vi "Test.vi"() -> ()   [LabVIEW 2014]
doc: "This VI is called when test mode begins, and will automatically be terminated when it ends. You can add manual or automatic tests and invoke them from the dashboard."
uses:
  <vilib>/Rock Robotics/WPI/RobotDrive/WPI_RobotDriveOpen2MotorWithTalon.vi
  <vilib>/Rock Robotics/SystemInterfaces/DIO/FPGA_DIOPWMChannel.ctl
  <vilib>/Rock Robotics/WPI/Joystick/WPI_JoystickDeviceEnum.ctl
panel:
  out "Distance":dbl
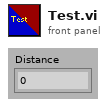
[diagram p1: front panel]
types:
  T1 = typedef "WPI_JoystickDevRef.ctl" = cluster{"Device":T2}
  T2 = typedef "WPI_JoystickDeviceEnum.ctl" = enum16{"USB 0", "USB 1", "USB 2", "USB 3", "USB 4", "USB 5"}
  T3 = typedef "FPGA_DIOPWMChannel.ctl" = enum8{"PWM 0", "PWM 1", "PWM 2", "PWM 3", "PWM 4", "PWM 5", "PWM 6", "PWM 7", "PWM 8", "PWM 9", "PWM MXP 0", "PWM MXP 1", "PWM MXP 2", "PWM MXP 3", "PWM MXP 4", "PWM MXP 5", "PWM MXP 6", "PWM MXP 7", "PWM MXP 8", "PWM MXP 9", "Invalid"}
  T4 = typedef "WPI_EncoderDevRef.ctl" = cluster{"DevStatus":errorcluster, "EncoderIndex":T5, "CounterIndex":T6, "DistancePerCount":dbl, "Decoding Type":T7}
  T5 = typedef "FPGA_EncoderIdx.ctl" = enum8{"Enc 0", "Enc 1", "Enc 2", "Enc 3", "Enc 4", "Enc 5", "Enc 6", "Enc 7", "Invalid"}
  T6 = typedef "FPGA_CounterCtrSystemIndex.ctl" = enum8{"Ctr 0", "Ctr 1", "Ctr 2", "Ctr 3", "Ctr 4", "Ctr 5", "Ctr 6", "Ctr 7", "Invalid"}
  T7 = typedef "WPI_EncoderType.ctl" = enum16{"1x", "2x", "4x"}
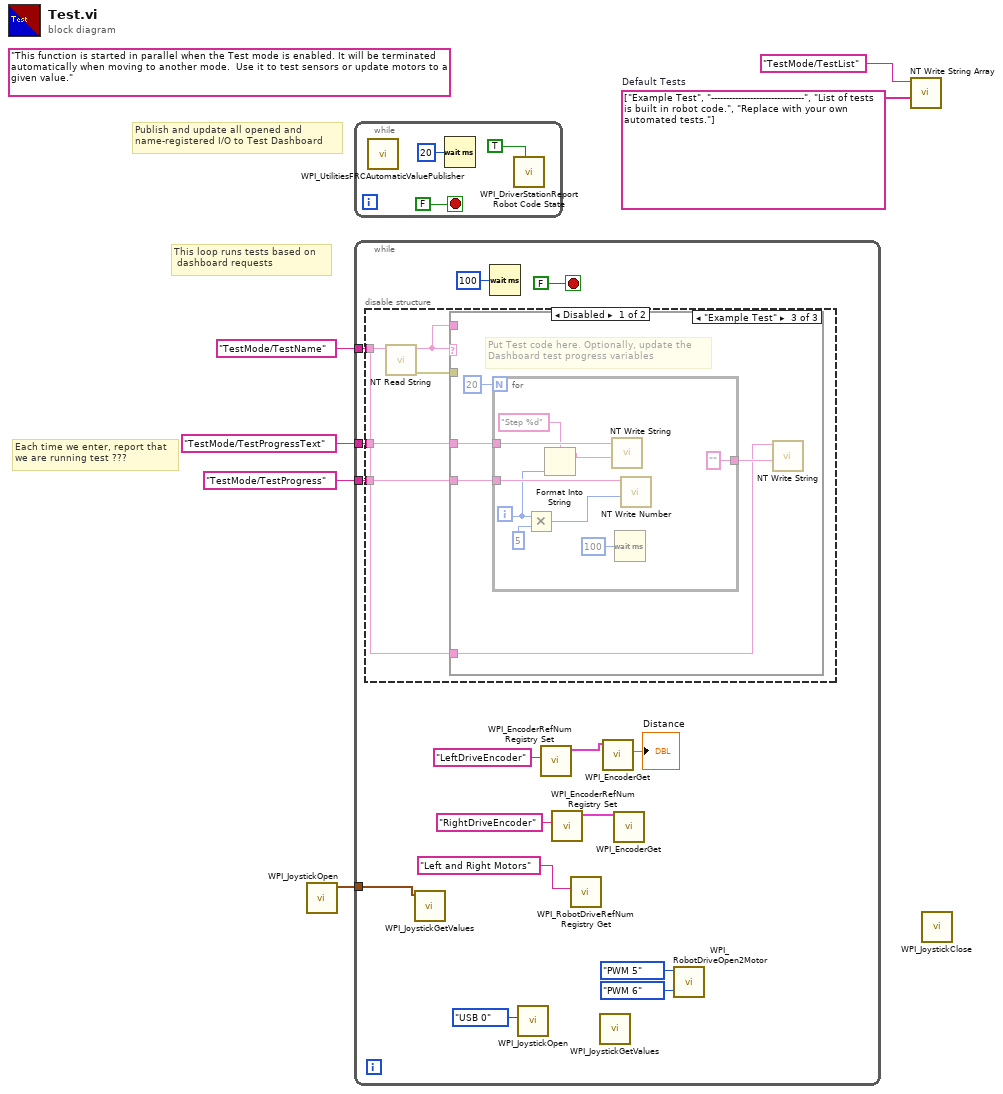
[diagram p0: block diagram]
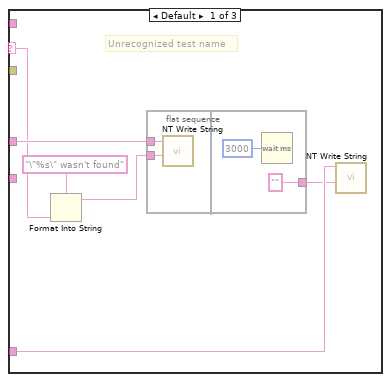
[diagram p2: hidden frame]
diagram:
  w3 = string[] ["Example Test", "-------------------------------", "List of tests is built in robot code.", "Replace with your own automated tests."]  # Default Tests
  (unwired) "This function is started in parallel when the Test mode is enabled. It will be terminated automatically when moving to another mode.  Use it to test sensors or update motors to a given value."
  # "This loop runs tests based on \n dashboard requests"
  # "Publish and update all opened and\nname-registered I/O to Test Dashboard"
  # "Each time we enter, report that\nwe are running test ???"
  n1 = call <vilib>:"WPI_JoystickOpen.vi"() -> ("JoystickDevRef"=w1:T1)  [unwired: 11 in]
  n2 = while {
    stop <- FALSE stop-if-true
    n3 = call <vilib>:"WPI_UtilitiesFRCAutomaticValuePublisher.vi"() -> ()  [unwired: 12 in]
    n4 = Wait (ms)(milliseconds to wait=u32 20) -> ()  [unwired: 1 out]
    n5 = call <vilib>:"WPI_DriverStationReport Robot Code State.vi"("Test"=TRUE ("Autonomous")) -> ()  [unwired: 10 in, 1 out]
  }
  n6 = while {
    tunnel: "TestMode/TestName" ("Name") -> [w20]
    tunnel: "TestMode/TestProgressText" ("Name") -> [w22]
    tunnel: "TestMode/TestProgress" ("Name") -> [w21]
    tunnel: w1 -> [w10]
    stop <- FALSE stop-if-true
    n7 = disable-structure shown="Disabled" {
      disable-tunnel: w22 -> [w29 _]
      disable-tunnel: w21 -> [w28 _]
      disable-tunnel: w20 -> [w26 _]
      frame Disabled {
        n8 = call <vilib>:"NT Read String.vi"("Name"=w26) -> ("error out"=w25:errorcluster, "String"=w27:string)  [unwired: 9 in]
        n9 = case shown="\"Example Test\"" w27 {
          selector: w27 -> [w34 _ _]
          tunnel: w26 -> [w31 _ w40]
          tunnel: w29 -> [w35 _ w43]
          tunnel: w28 -> [_ _ w44]
          tunnel: w27 -> [_ _ _]
          tunnel: w25 -> [_ _ _]
          frame Default {
            # "Unrecognized test name"
            n10 = Format Into String(format string="\"%s\" wasn't found" ("Name"), w34) -> (resulting string=w33:string)  [unwired: 2 in, 1 out]
            n11 = flat-sequence {
              tunnel: w35 -> [w36]
              tunnel: w33 -> [w37]
              tunnel: ["" ("Name")] -> w30
              frame #0 {
                n12 = call <vilib>:"NT Write String.vi"("String"=w37, "Name"=w36) -> ()  [unwired: 9 in, 1 out]
              }
              frame #1 {
                n13 = Wait (ms)(milliseconds to wait=u32 3000) -> ()  [unwired: 1 out]
              }
            }
            n14 = call <vilib>:"NT Write String.vi"("String"=w30, "Name"=w31) -> ()  [unwired: 9 in, 1 out]
          }
          frame "" {
            # "No test to run"
          }
          frame "Example Test" {
            # "Put Test code here. Optionally, update the\nDashboard test progress variables"
            n15 = for {
              N: 20 -> [_]
              tunnel: w44 -> [w53]
              tunnel: w43 -> [w51]
              tunnel: ["" ("String")] -> w41
              i -> [w48]
              n16 = Multiply(x=w48, y=u32 5 ("milliseconds to wait")) -> (x*y=w49:u32)
              n17 = Format Into String(format string="Step %d", w48) -> (resulting string=w46:string)  [unwired: 2 in, 1 out]
              n18 = call <vilib>:"NT Write String.vi"("String"=w46, "Name"=w51) -> ()  [unwired: 9 in, 1 out]
              n19 = Wait (ms)(milliseconds to wait=u32 100) -> ()  [unwired: 1 out]
              n20 = call <vilib>:"NT Write Number.vi"("Numeric"=w49, "Name"=w53) -> ()  [unwired: 9 in, 1 out]
            }
            n21 = call <vilib>:"NT Write String.vi"("String"=w41, "Name"=w40) -> ()  [unwired: 9 in, 1 out]
          }
        }
      }
      frame Enabled {
      }
    }
    n22 = call <vilib>:"WPI_JoystickGetValues.vi"("JoystickDevRef"=w10) -> ()  [unwired: 6 in, 5 out]
    n23 = Wait (ms)(milliseconds to wait=u32 100) -> ()  [unwired: 1 out]
    n24 = call <vilib>:"WPI_JoystickOpen.vi"("JoystickDevice"=WPI_JoystickDeviceEnum."USB 0") -> ()  [unwired: 10 in, 1 out]
    n25 = call <vilib>:"WPI_EncoderRefNum Registry Set.vi"("refnum name"="LeftDriveEncoder") -> ("EncoderDevRef"=w15:T4)  [unwired: 9 in, 1 out]
    n26 = call <vilib>:"WPI_EncoderRefNum Registry Set.vi"("refnum name"="RightDriveEncoder") -> ("EncoderDevRef"=w16:T4)  [unwired: 9 in, 1 out]
    n27 = call <vilib>:"WPI_RobotDriveRefNum Registry Get.vi"("refnum name"="Left and Right Motors") -> ()  [unwired: 9 in, 2 out]
    n28 = call <vilib>:"WPI_JoystickGetValues.vi"() -> ()  [unwired: 7 in, 5 out]
    n29 = call <vilib>:"WPI_EncoderGet.vi"("EncoderDevRef"=w15) -> ("Distance"=→"Distance":dbl)  [unwired: 5 in, 5 out]
    n30 = call <vilib>:"WPI_EncoderGet.vi"("EncoderDevRef"=w16) -> ()  [unwired: 5 in, 6 out]
    n31 = call-poly <vilib>:"WPI_RobotDriveOpen2Motor.vi"("Right Motor"=FPGA_DIOPWMChannel."PWM 6", "Left Motor"=FPGA_DIOPWMChannel."PWM 5") -> ()  [unwired: 8 in, 2 out]
  }
  n32 = call <vilib>:"NT Write String Array.vi"("String Array"=w3, "Name"="TestMode/TestList") -> ()  [unwired: 9 in, 1 out]
  n33 = call <vilib>:"WPI_JoystickClose.vi"() -> ()  [unwired: 12 in]
